vi "RSNRPZ Set Scope Average Count.vi"(8 "error in (no error)":errorcluster, 9 "Count (4)":i32=4, 10 "Channel (1)":i32=1, 11 "VISA session":refnum<visa-resource-name> caption="VISA resource name") -> (0 "error out":errorcluster, 3 "dup VISA session":refnum<visa-resource-name> caption="VISA resource name")   [LabVIEW 2019]
doc: "This VI sets the length of the filter for the Scope mode. The wider the filter the lower the noise and the longer it takes to obtain a measured value.\n\nRemote-control command(s):\nSENS:TRAC:AVER:COUN"
uses:
  rsnrpz_32.dll
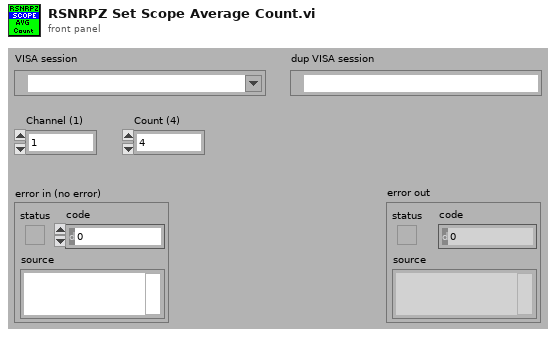
[diagram p1: front panel]
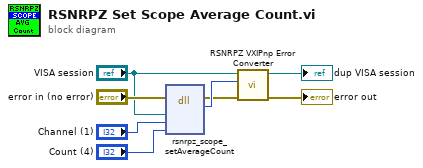
[diagram p0: block diagram]
diagram:
  n1 = dll-call lib="C:/Users/LABadmin/Documents/Jarvis/user_lib/rsnrpz/rsnrpz_32.dll" fn="rsnrpz_scope_setAverageCount"(error in="error in (no error)", "VISA Session"="VISA session", "Channel"="Channel (1)", "Count"="Count (4)") -> (error out=w5:errorcluster, "Status"=w8:i32)  [unwired: 5 in, 1 out]
  n2 = call <instrlib>:"RSNRPZ VXIPnp Error Converter.vi"("error in"=w5, "VXIPnp error code"=w8, "VISA session"="VISA session") -> ("error out"=→"error out":errorcluster, "dup VISA session"=→"dup VISA session":refnum<visa-resource-name>)  [unwired: 7 in]
